vi "MQTT_PUBLISH.vi"(6 "MENSAJE":string, 7 "SEND":bool, 8 "error IN":errorcluster, 9 "TOPIC":string, 10 "IP":string, 11 "VISA resource name IN":refnum<visa-resource-name>) -> (0 "error out":errorcluster, 1 "read buffer":string, 3 "VISA resource name out":refnum<visa-resource-name>)   [LabVIEW 2025]
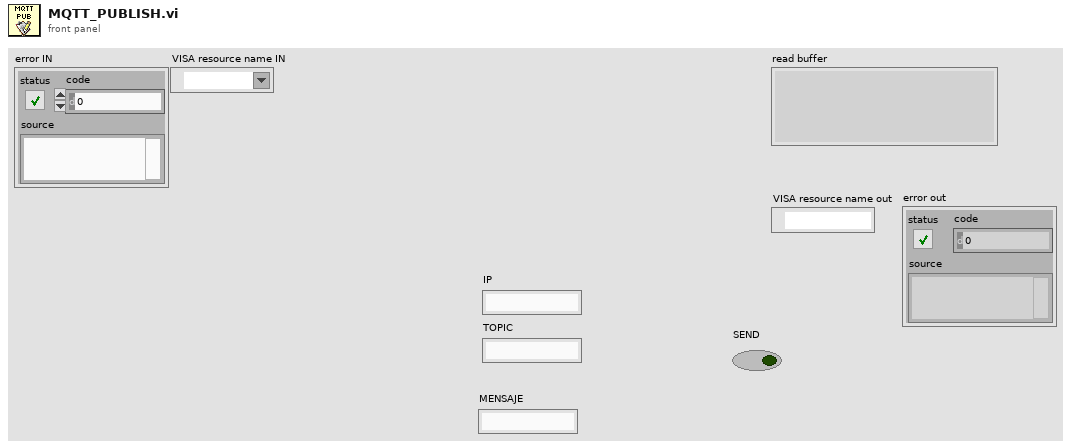
[diagram p1: front panel]
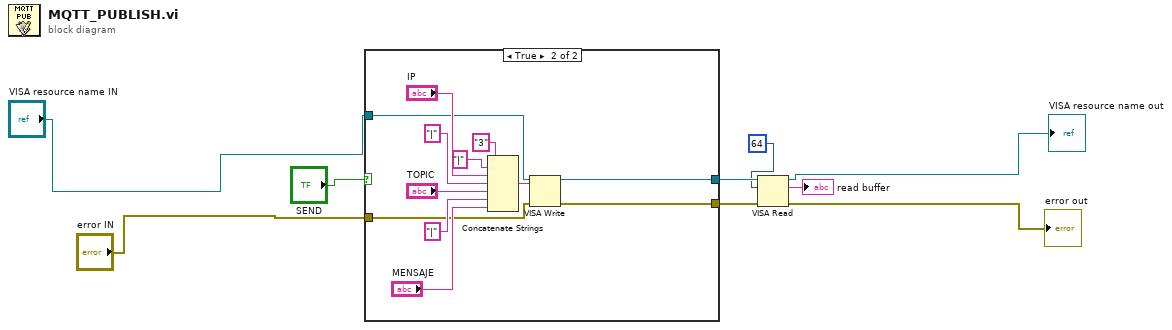
[diagram p0: block diagram]
diagram:
  n1 = case shown="True" "SEND" {
    tunnel: "VISA resource name IN" -> [w11 w17]
    tunnel: "error IN" -> [w10 w16]
    tunnel: [w10 w13] -> w5
    tunnel: [w11 w12] -> w4
    frame False {
    }
    frame True {
      n2 = Concatenate Strings("3", "|", "IP", "|", "TOPIC", "|", "MENSAJE") -> (w18:string)
      n3 = VISA Write(VISA resource name=w17, write buffer=w18, error in (no error)=w16) -> (VISA resource name out=w12:refnum<visa-resource-name>, error out=w13:errorcluster)  [unwired: 1 out]
    }
  }
  n4 = VISA Read(VISA resource name=w4, byte count=u32 64, error in (no error)=w5) -> (VISA resource name out=→"VISA resource name out":refnum<visa-resource-name>, read buffer=→"read buffer":string, error out=→"error out":errorcluster)  [unwired: 1 out]
